vi "Read Measurements.vi"(7 "Channel (1: 1)":i32(ring)=1 items=["SIM900", "1", "2", "3", "4", "5", "6", "7", "8", "9", "A", "B", "C", "D"], 8 "error in (no error)":errorcluster, 10 "Number of Samples (1)":i32=1, 11 "VISA resource name":refnum<visa-resource-name>) -> (0 "error out":errorcluster, 1 "Amplified Error":dbl[](array[numeric]), 2 "Measure Input":dbl[](array[numeric]), 3 "VISA resource name out":refnum<visa-resource-name>, 4 "Output":dbl[](array[numeric]), 5 "Setpoint":dbl[](array[numeric]))   [LabVIEW 2019, in "Stanford Research SIM900 Series.lvlib"]
doc: "Reads the specified number of samples of the Setpoint, Measure Input, Amplified Error and Output from the SIM960 module. Measurments are taken at a rate of about half a second per measurment. If a large number of samples are requested this VI will take a long time to execute.\n\n<b>Note:</b>\nThis VI only applies to the SIM960 module."
uses:
  Stanford Research SIM900 Series.lvlib
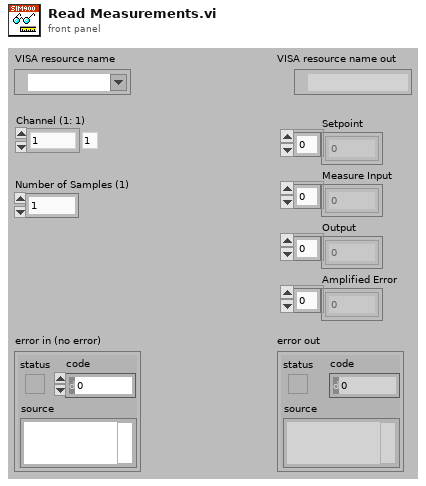
[diagram p1: front panel]
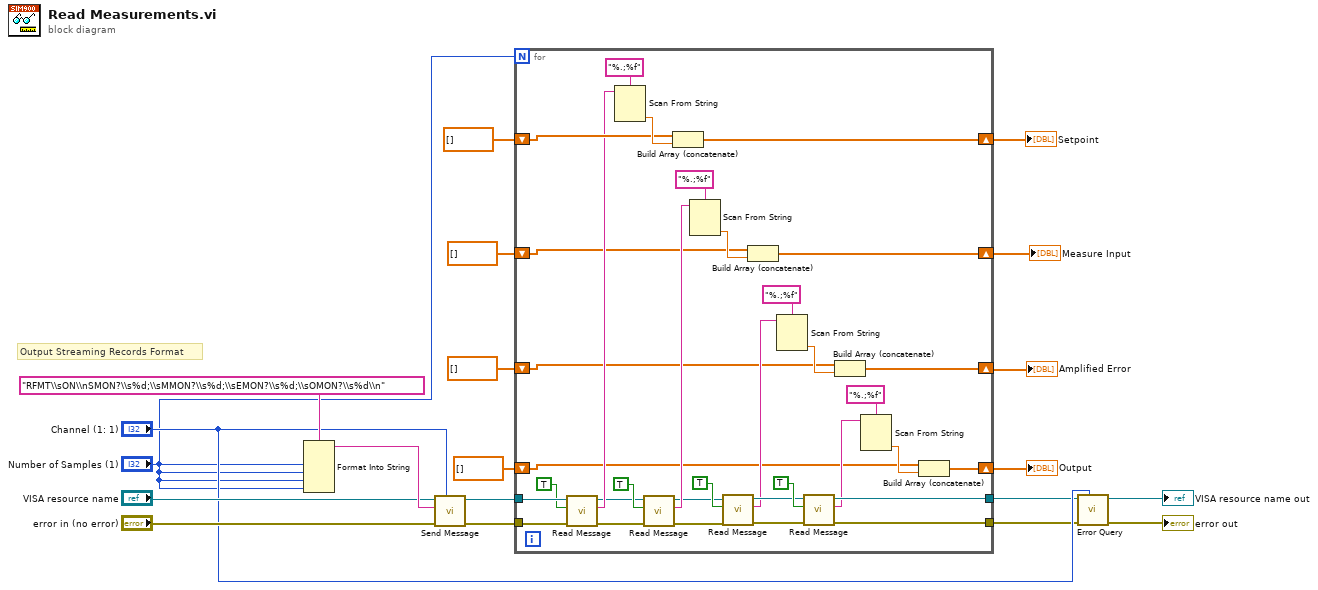
[diagram p0: block diagram]
diagram:
  # "Output Streaming Records Format"
  n1 = Format Into String(format string="RFMT\\sON\\nSMON?\\s%d;\\sMMON?\\s%d;\\sEMON?\\s%d;\\sOMON?\\s%d\\n", "Number of Samples (1)", "Number of Samples (1)", "Number of Samples (1)", "Number of Samples (1)") -> (resulting string=w16:string)  [unwired: 2 in, 1 out]
  n2 = call "Send Message.vi"("Channel (0: SIM900)"="Channel (1: 1)", "error in (no error)"="error in (no error)", "Message (\"\")"=w16, "VISA resource name"="VISA resource name") -> ("error out"=w17:errorcluster, "VISA resource name out"=w18:refnum<visa-resource-name>)  [unwired: 6 in]
  n3 = for {
    N: "Number of Samples (1)" -> [_]
    tunnel: w18 -> [w50]
    tunnel: w17 -> [w49]
    shift-right: [w52] -> w10
    shift-left: dbl[] [] -> [w51]
    tunnel: [w34] -> w9
    tunnel: [w33] -> w8
    shift-right: [w31] -> w6
    shift-left: dbl[] [] -> [w32]
    shift-right: [w26] -> w3
    shift-left: dbl[] [] -> [w27]
    shift-right: [w21] -> w2
    shift-left: dbl[] [] -> [w22]
    n4 = call "Read Message.vi"("error in (no error)"=w49, "Enable Header Information (False)"=TRUE ("From Port"), "VISA resource name"=w50) -> ("error out"=w42:errorcluster, "Message"=w48:string, "VISA resource name out"=w43:refnum<visa-resource-name>)  [unwired: 6 in]
    n5 = Scan From String(format string="%.;%f", input string=w48) -> (output 1=w54:dbl)  [unwired: 3 in, 3 out]
    n6 = call "Read Message.vi"("error in (no error)"=w42, "Enable Header Information (False)"=TRUE ("From Port"), "VISA resource name"=w43) -> ("error out"=w38:errorcluster, "Message"=w41:string, "VISA resource name out"=w39:refnum<visa-resource-name>)  [unwired: 6 in]
    n7 = Build Array (concatenate)(w51, w54) -> (w52:dbl[])
    n8 = Scan From String(format string="%.;%f", input string=w41) -> (output 1=w46:dbl)  [unwired: 3 in, 3 out]
    n9 = call "Read Message.vi"("error in (no error)"=w38, "Enable Header Information (False)"=TRUE ("From Port"), "VISA resource name"=w39) -> ("error out"=w35:errorcluster, "Message"=w28:string, "VISA resource name out"=w36:refnum<visa-resource-name>)  [unwired: 6 in]
    n10 = Build Array (concatenate)(w32, w46) -> (w31:dbl[])
    n11 = Scan From String(format string="%.;%f", input string=w28) -> (output 1=w30:dbl)  [unwired: 3 in, 3 out]
    n12 = call "Read Message.vi"("error in (no error)"=w35, "Enable Header Information (False)"=TRUE ("From Port"), "VISA resource name"=w36) -> ("error out"=w33:errorcluster, "Message"=w23:string, "VISA resource name out"=w34:refnum<visa-resource-name>)  [unwired: 6 in]
    n13 = Build Array (concatenate)(w27, w30) -> (w26:dbl[])
    n14 = Scan From String(format string="%.;%f", input string=w23) -> (output 1=w24:dbl)  [unwired: 3 in, 3 out]
    n15 = Build Array (concatenate)(w22, w24) -> (w21:dbl[])
  }
  "Amplified Error" <- w3
  "Setpoint" <- w10
  "Measure Input" <- w6
  "Output" <- w2
  n16 = call "Error Query.vi"("Channel (0: SIM900)"="Channel (1: 1)", "error in (no error)"=w8, "VISA resource name"=w9) -> ("error out"=→"error out":errorcluster, "VISA resource name out"=→"VISA resource name out":refnum<visa-resource-name>)  [unwired: 5 in, 2 out]
